vi "LeadLagDiffEqn.vi"(6 "Enable?":bool, 8 "c":fxp<+/-,24,5>, 9 "b":fxp<+/-,24,5>, 10 "a":fxp<+/-,24,1>, 11 "Input":fxp<+/-,18,5>) -> (3 "Output":fxp<+/-,18,5>)   [LabVIEW 2019, in "FPGA functions.lvlib"]
doc: "Implement a first order difference equation of the form:\ny(k) = a*y(k-1) + b*u(k) - c*u(k-1)\n\nY/U = (bz-c)/(z-a)"
uses:
  FPGA functions.lvlib
  <vilib>/Platform/TimedLoop/XDataNode/timing_clust.ctl
  <vilib>/Platform/TimedLoop/XDataNode/nitl_modes.ctl
  <vilib>/Platform/TimedLoop/XDataNode/wakeup.ctl
  <vilib>/Platform/TimedLoop/XDataNode/XDataNode.xnode
  <vilib>/rvi/FXPMathLib/basic elements/FxpDiscreteDelay/XNode/nifxpmath_DiscreteDelay.xnode
  <vilib>/rvi/FXPMathLib/FxpMul/XNode/nifxpmath_Multiplier.xnode
  <vilib>/rvi/FXPMathLib/FxpAdd/XNode/nifxpmath_Add.xnode
  <vilib>/rvi/FXPMathLib/FxpSub/XNode/nifxpmath_Sub.xnode
  <vilib>/Platform/TimedLoop/XDataNode/XDNodeRunTimeDep.lvlib
  <vilib>/rvi/FXPMathLib/sim/FxpSim.dll
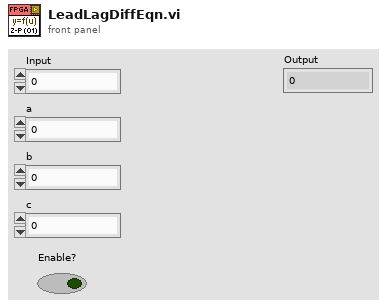
[diagram p1: front panel]
types:
  T1 = typedef "XDNodeRunTimeDep.lvlib/timing_clust.ctl" = cluster{"Expected End [f-1]":u64, "Actual End [f-1]":u64, "Finished Late? [f-1]":bool, "Expected End [i-1]":u64, "Actual End [i-1]":u64, "Finished Late? [i-1]":bool, "Expected Start [i]":u64, "Actual Start [i]":u64, "Expected Start [f]":u64, "Actual Start [f]":u64, "Source Name":string, "Structure Name":string, "Period":i64, "Deadline":i64, "Offset":i64, "Start":i64, "Priority":i32, "Timeout":i32, "Mode":T2, "Wakeup Reason":T3, "Error":errorcluster, "Source Type":string, "Secondary Source Type":string, "Global End Time":u64, "Global Start Time":u64, "Frame Duration":u64, "Iteration Duration":u64, "Assigned CPU":i32, "I/O Scan Engine Mode":u32}
  T2 = typedef "XDNodeRunTimeDep.lvlib/nitl_modes.ctl" = enum32{"No Change", "Process missed periods, maintain original phase", "Discard missed periods, maintain original phase", "Process missed periods, ignore original phase", "Discard missed periods, ignore original phase"}
  T3 = typedef "XDNodeRunTimeDep.lvlib/wakeup.ctl" = enum32{"Normal", "Aborted", "Asynchronous wakeup", "Timing source error", "Timed loop error", "Timeout"}
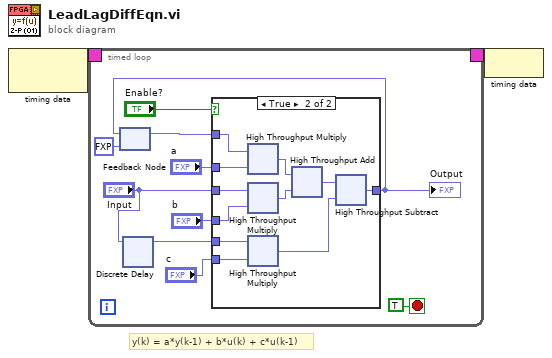
[diagram p0: block diagram]
diagram:
  # "y(k) = a*y(k-1) + b*u(k) + c*u(k-1)"
  n1 = node-c288() -> (w2:T1)  [unwired: 1 in]
  n2 = timed-loop {
    timing: w2 -> [_]
    timing-out: [_] -> w1
    stop <- TRUE stop-if-true
    n3 = feedback #1(fxp<+/-,18,5> 0.0 ("x+y")) -> (w7:fxp<+/-,18,5>)
    n4 = xnode ("Discrete Delay")("D"="Input") -> ("Q"=w5:fxp<+/-,18,5>)
    n5 = case shown="True" "Enable?" {
      tunnel: "Input" -> [w13 w24]
      tunnel: "a" -> [_ w21]
      tunnel: [w13 w23] -> w9
      tunnel: w7 -> [_ w22]
      tunnel: w5 -> [_ w19]
      tunnel: "b" -> [_ w20]
      tunnel: "c" -> [_ w18]
      frame False {
      }
      frame True {
        n6 = xnode ("High Throughput Multiply")("x"=w22, "y"=w21) -> ("x*y"=w16:fxp<+/-,18,5>)
        n7 = xnode ("High Throughput Multiply")("x"=w24, "y"=w20) -> ("x*y"=w15:fxp<+/-,18,5>)
        n8 = xnode ("High Throughput Multiply")("x"=w19, "y"=w18) -> ("x*y"=w17:fxp<+/-,18,5>)
        n9 = xnode ("High Throughput Add")("x"=w16, "y"=w15) -> ("x+y"=w14:fxp<+/-,19,6>)
        n10 = xnode "High Throughput Subtract"("x"=w14, "y"=w17) -> ("x-y"=w23:fxp<+/-,18,5>)
      }
    }
    "Output" <- w9
    n11 = feedback-in #1(w9) -> ()
  }
  n12 = node-c288(w1) -> ()
